vi "COMMAND_LONG.vi"(8 "Target System and Target Component":u8=1, 9 "Mission Params":u8[](array[numeric]), 10 "Confirmation":u8, 11 "Command ID":u16) -> (3 "MAVLink Message":u8[](array[numeric]))   [LabVIEW 2014]
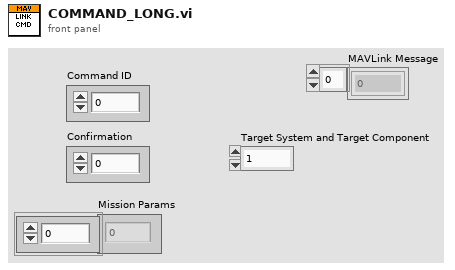
[diagram p1: front panel]
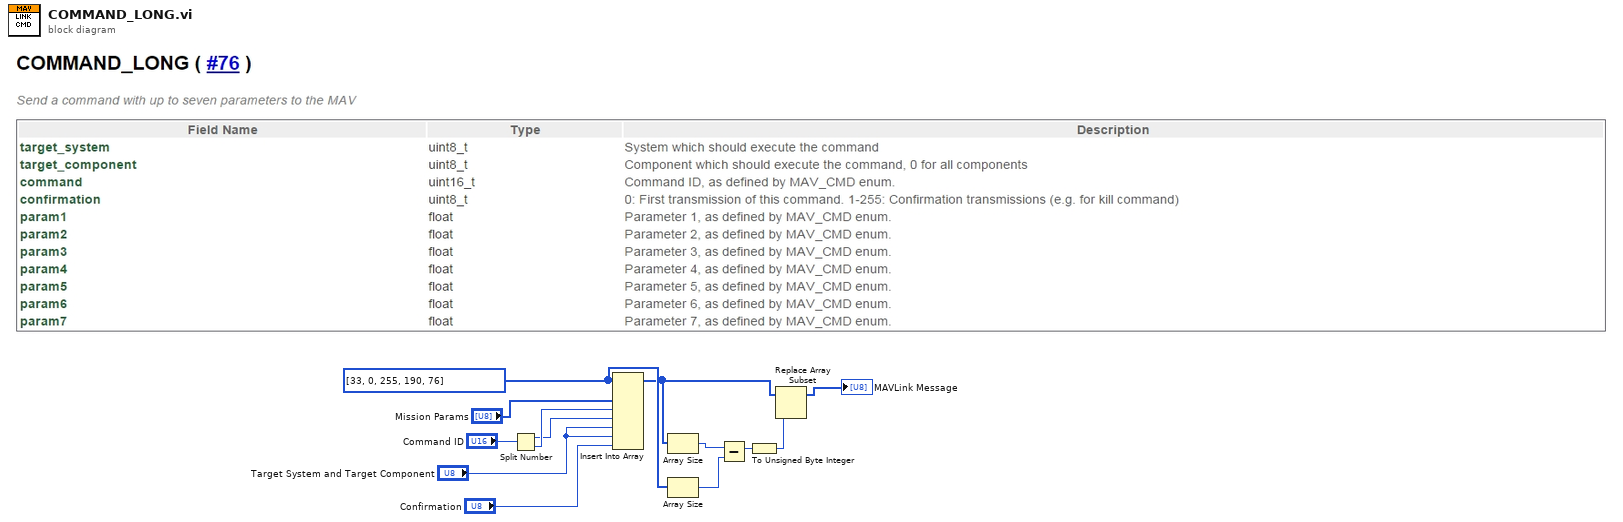
[diagram p0: block diagram]
diagram:
  w7 = u8[] [33, 0, 255, 190, 76]
  n1 = Split Number(x="Command ID") -> (hi(x)=w10:u8, lo(x)=w11:u8)
  n2 = Insert Into Array(array=w7, new element #1="Mission Params", new element #2=w11, new element #3=w10, new element #4="Target System and Target Component", new element #5="Target System and Target Component", new element #6="Confirmation") -> (w5:u8[])  [unwired: 1 in]
  n3 = Array Size(array=w5) -> (size(s)=w8:i32)
  n4 = Array Size(array=w7) -> (size(s)=w6:i32)
  n5 = Subtract(x=w8, y=w6) -> (x-y=w3:i32)
  n6 = To Unsigned Byte Integer(number=w3) -> (unsigned 8bit integer=w2:u8)
  n7 = Replace Array Subset(array=w5, new element=w2) -> (→"MAVLink Message":u8[])  [unwired: 1 in]
